vi "Offset Locking and Active Slave Locking v3.2.vi"() -> ()   [LabVIEW 2018]
uses:
  <vilib>/Utility/error.llb/DialogType.ctl
  <vilib>/Analysis/1siggen.llb/Ramp Pattern by Samples.vi
  <vilib>/measure/mamon.llb/Waveform Peak Detection for 1 Chan.vi
  <vilib>/addons/control/pid/pid.llb/PID Advanced (DBL).vi
  <vilib>/measure/NI_MAPro.lvlib
  <vilib>/addons/control/pid/NI_PID_pid.lvlib
  <vilib>/Analysis/NI_AALBase.lvlib
  <vilib>/measure/NI_MABase.lvlib
panel:
  in  "Drift Threshold":dbl
  out "Waveform Chart":dbl(graph)
  out "Slave Current Adj":dbl
  out "Master-Slave Peak Height":dbl
  in  "Locked Peak Height Min":dbl
  in  "Active Slave Lock On":bool
  in  "Slave Current Adjust":dbl
  out "Target \nPeak":dbl
  out "Calibration\n Peaks":dbl[](array[numeric])
  in  "Minimum \namplitude\nfor Calibration":dbl=2.1 format="%#_13g V"
  in  "width":i32=1000
  in  "start":dbl format="%0.2f"
  in  "end":dbl=1.0 format="%0.2f"
  in  "samples":i32=128
  in  "Waveform Test?":bool
  in  "reset signal":bool
  in  "phase":dbl format="%.2p"
  out "Chirp Rate":dbl format="%#_g GHz/ms"
  out "Single Mode?":bool
  out "# of Peaks found when Chirping?":i32
  in  "Minimum amplitude for Slave":dbl=0.15 format="%.2p"
  in  "Minimum \namplitude\nfor peaks":dbl=1.2 format="%#_13g V"
  in  "PZT Voltage to \nFrequency Conversion":dbl=-1.41655 format="%#_g V/GHz"
  out "PZT Chirp Output":waveform(dbl)(graph)
  in  "offset":dbl format="%0.2p V"
  in  "Sampling Info":cluster{"Fs":dbl, "#s":dbl}={"Fs"=10000.0, "#s"=100.0} {"Fs" format="%.2p"}
  in  "frequency":dbl=10.0 format="%0.2p Hz"
  in  "Chirp Amplitude":dbl=1.5 format="%0.2p GHz"
  in  "Run Chirp Program?":bool
  out "Run Time (min)":dbl
  out "standard deviation":dbl format="%0.3e"
  out "# found":i32
  out "Offset":dbl(graph)
  in  "Manual PZT Control":dbl format="%#_g V"
  in  "Engage PZT PID?":bool
  out "Offset (GHz)":dbl format="%#_4g"
  in  "# of Shots for Averaging":i32=100
  in  "Name Convention":string="Chirp Offset Lock Log"
  in  "Save Directory":path=path "C:/Users/LabUser/Google Drive/Measurements/04-2018"
  out "Enough\n peaks?":bool
  out "PZT Output":dbl(graph)
  in  "PID Gains":T1={"proportional gain (Kc)"=-1.0, "integral time (Ti, min)"=0.01, "derivative time (Td, min)"=0.0} {"derivative time (Td, min)" format="%.3f"; "integral time (Ti, min)" format="%.3f"; "proportional gain (Kc)" format="%.3f"}
  out "dt out (s)":dbl format="%.3f"
  in  "Frequency Offset Setpoint (GHz)":dbl=4.0 format="%.3f"
  out "GHz/sec":dbl
  out "dt":dbl format="%#_4g"
  out "Locations":dbl[](array[numeric]) format="%.2p"
  out "Amplitudes":dbl[](array[numeric]) format="%.2p"
  out "2nd Derivatives":dbl[](array[numeric]) format="%.2p"
  out "10 GHz FPI":dynamicdata(graph)
  in  "Stop":bool
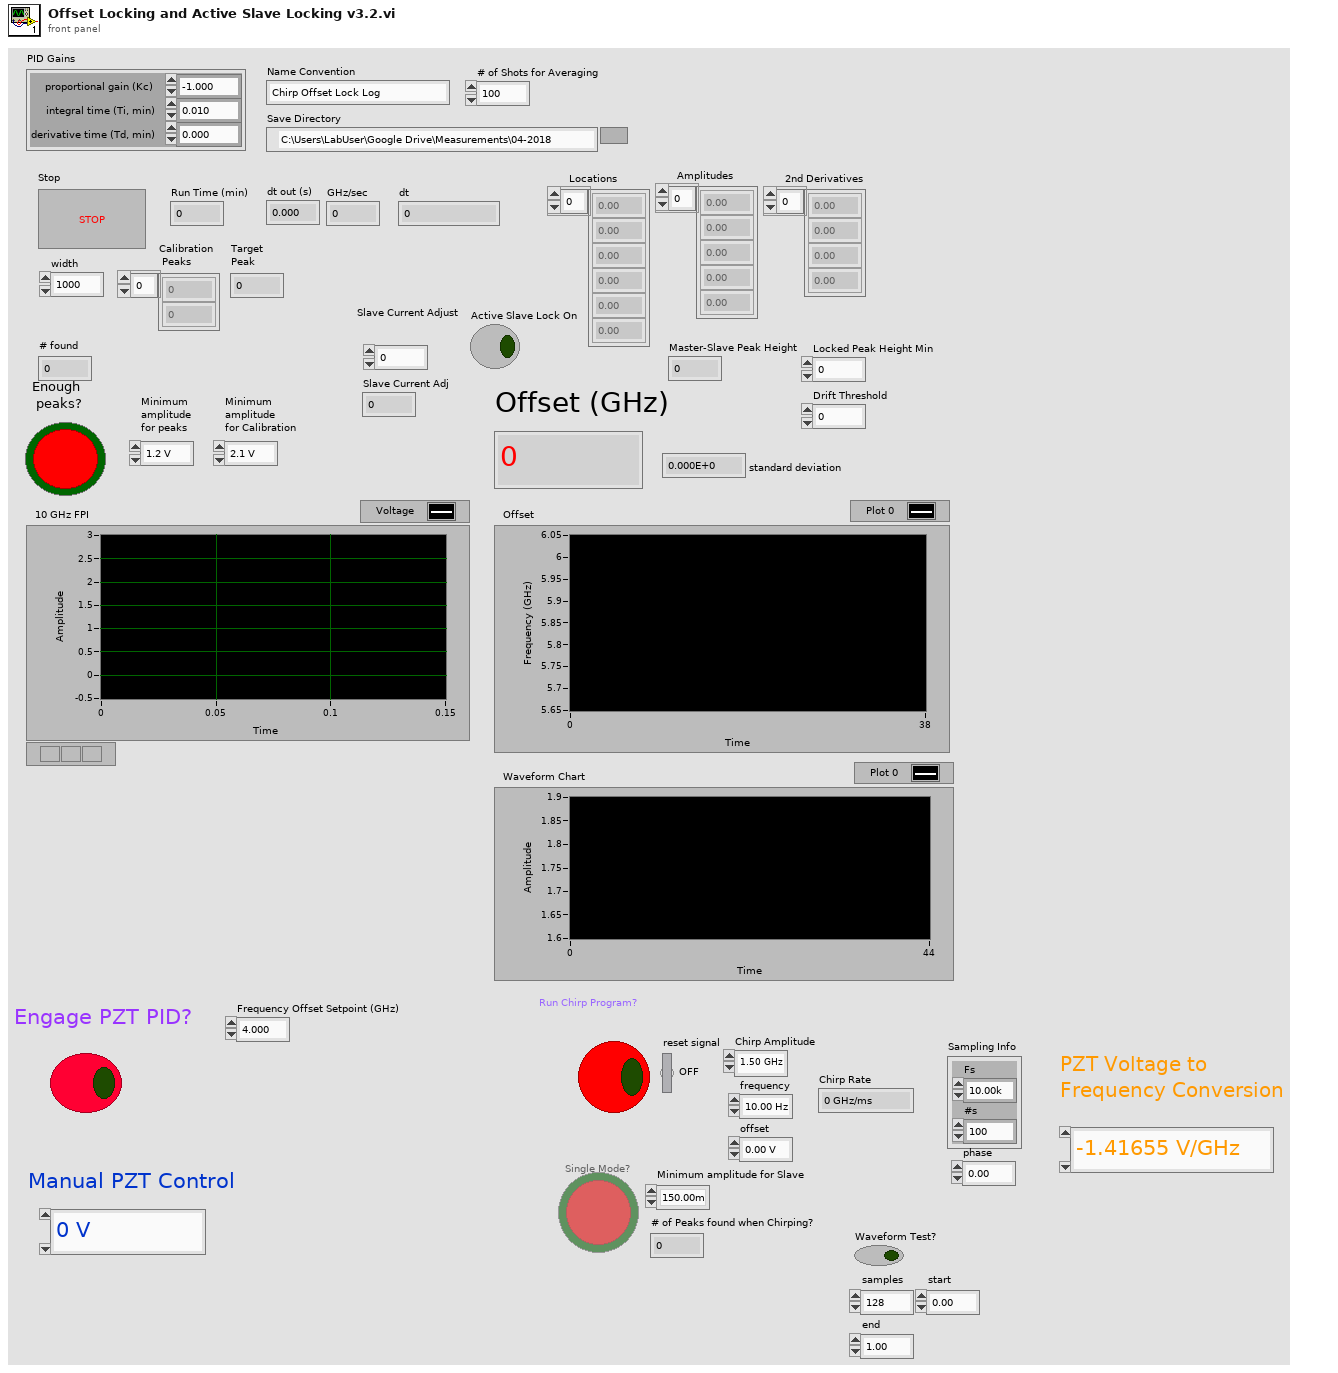
[diagram p1: front panel]
types:
  T1 = cluster{"proportional gain (Kc)":dbl, "integral time (Ti, min)":dbl, "derivative time (Td, min)":dbl}
  T2 = enum8{"Enabled", "Disabled", "Disabled and Grayed Out"}
  T3 = typedef "DialogType.ctl" = u16
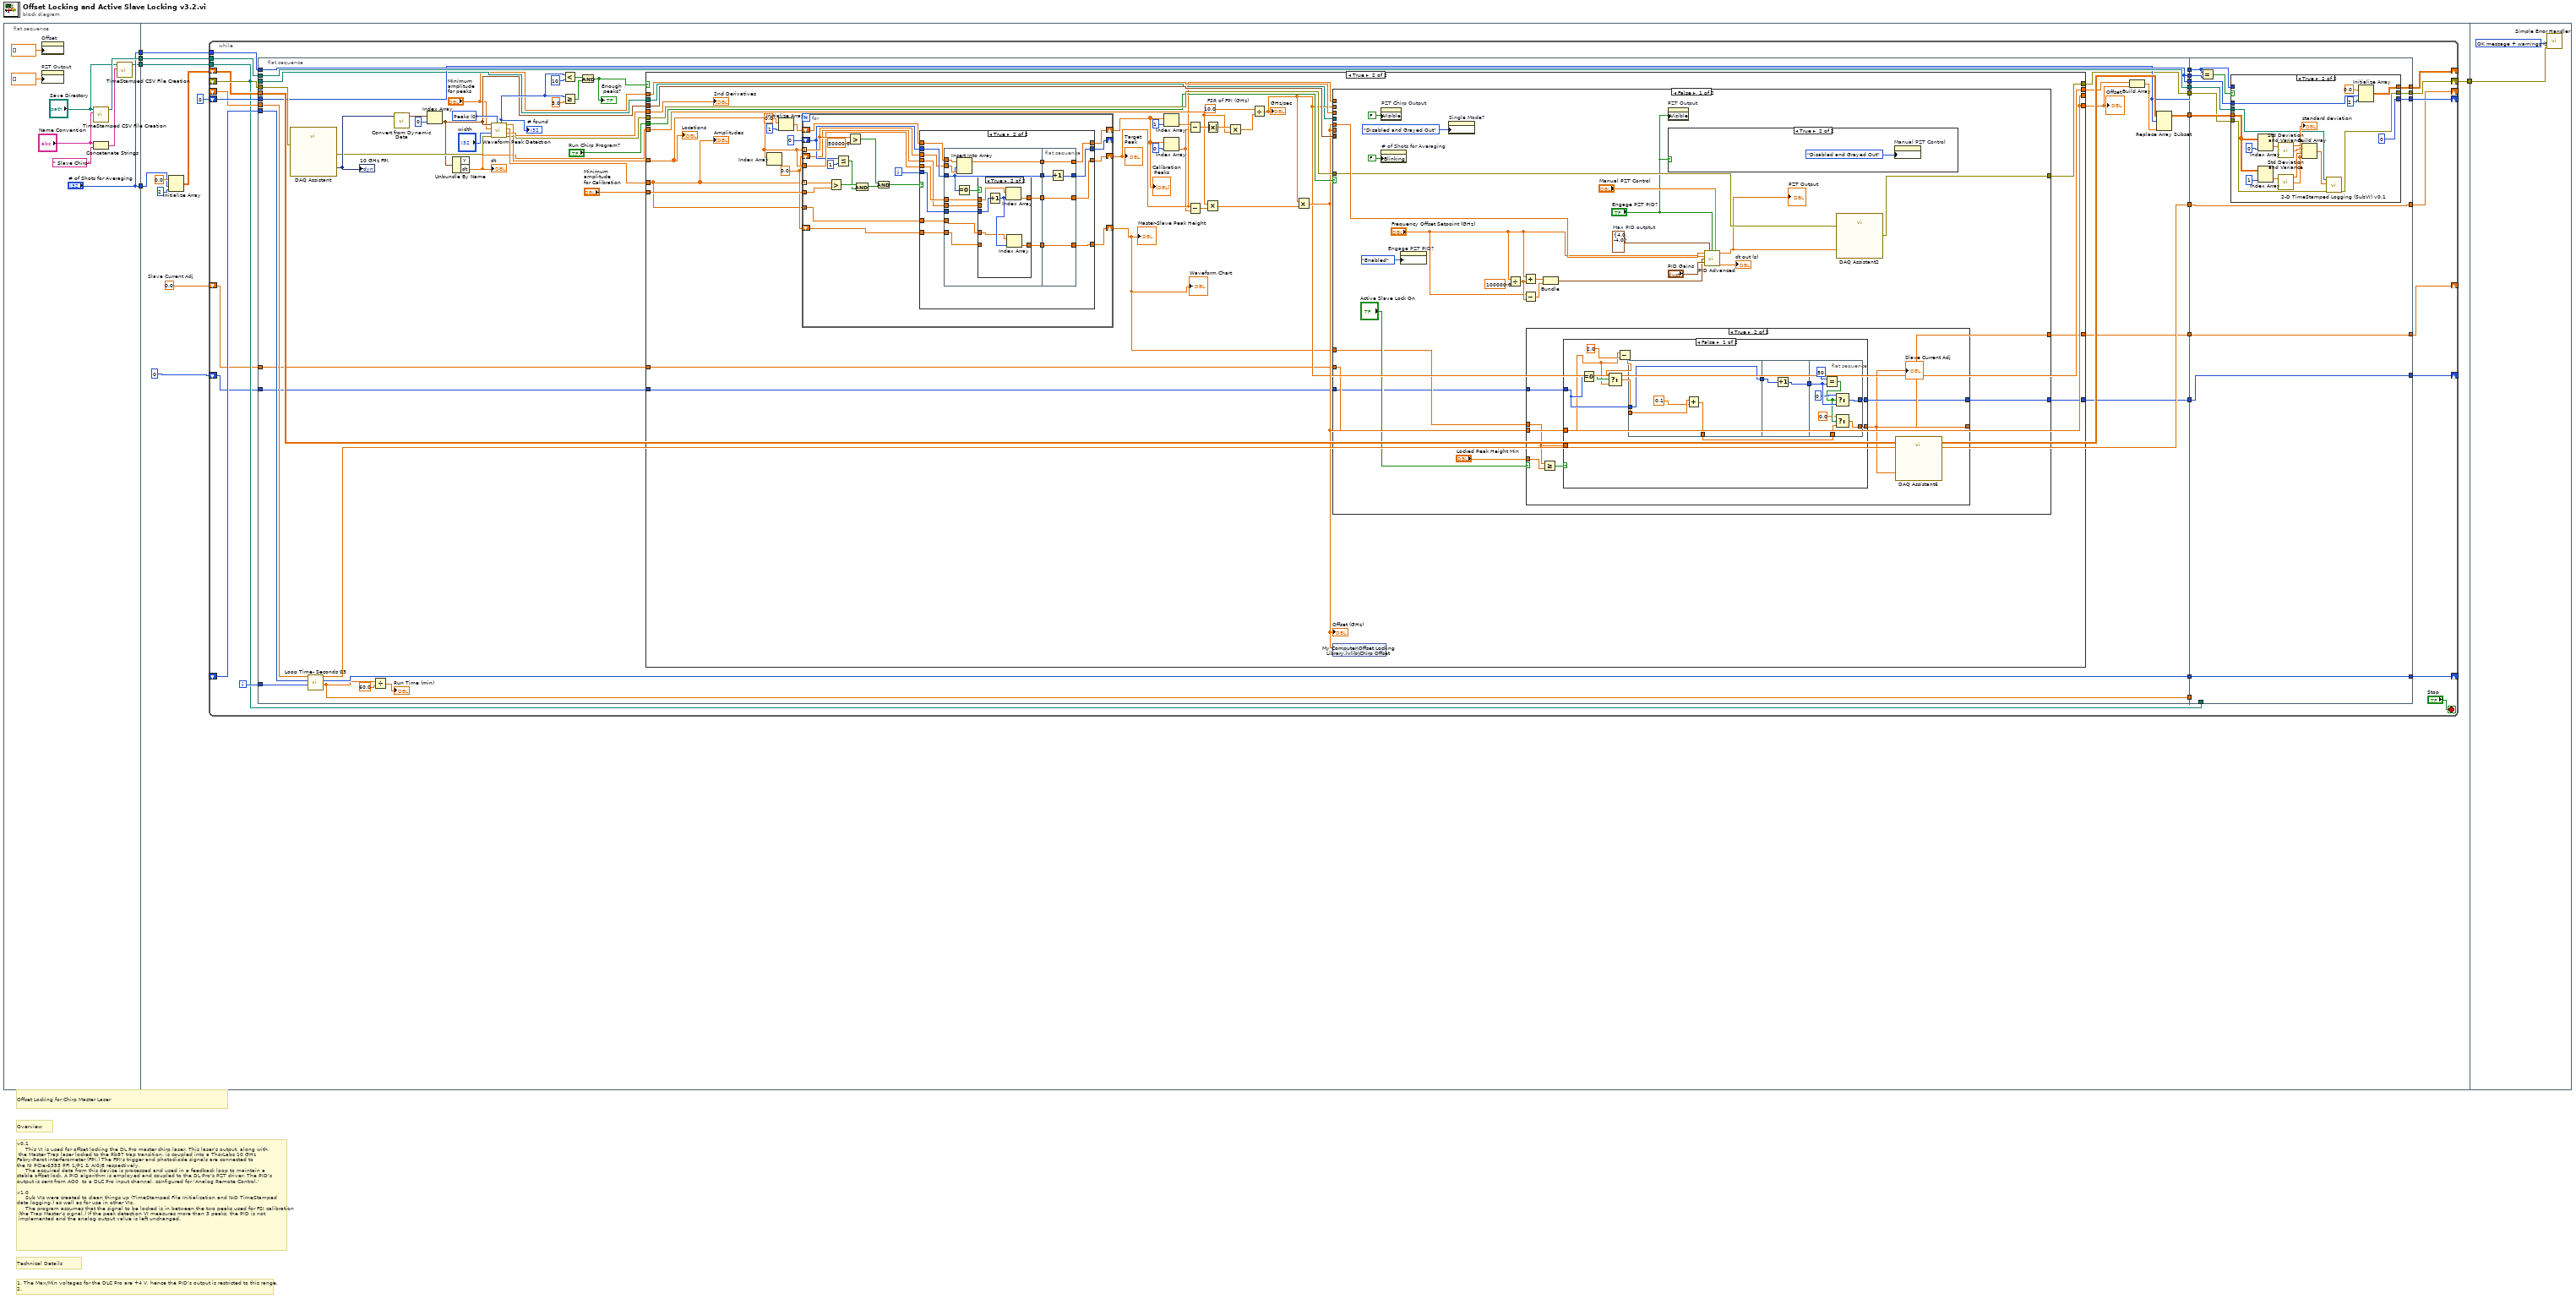
[diagram p0: block diagram]
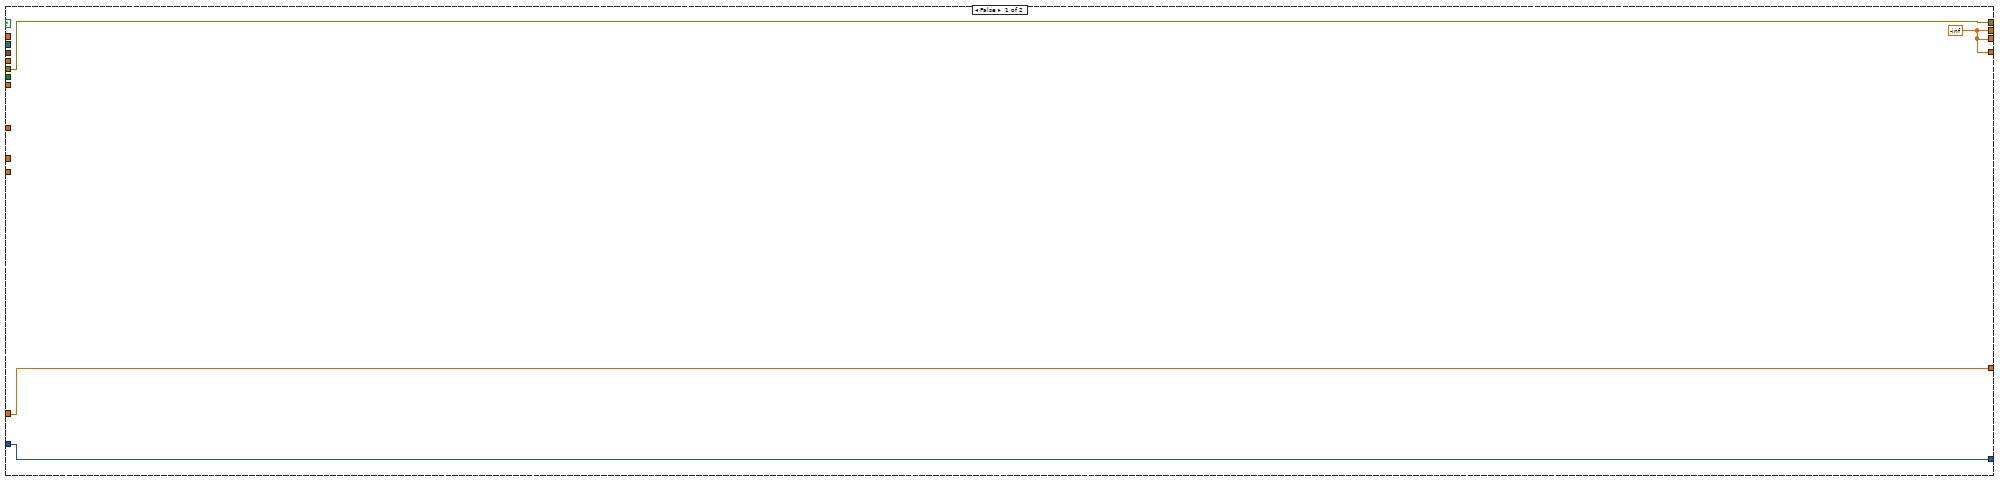
[diagram p2: hidden frame]
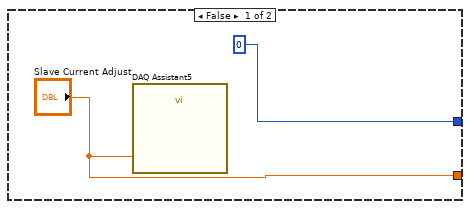
[diagram p5: hidden frame]
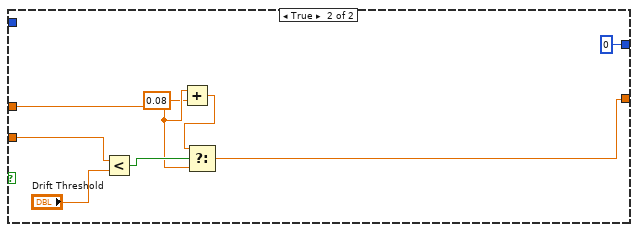
[diagram p6: hidden frame]
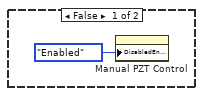
[diagram p7: hidden frame]
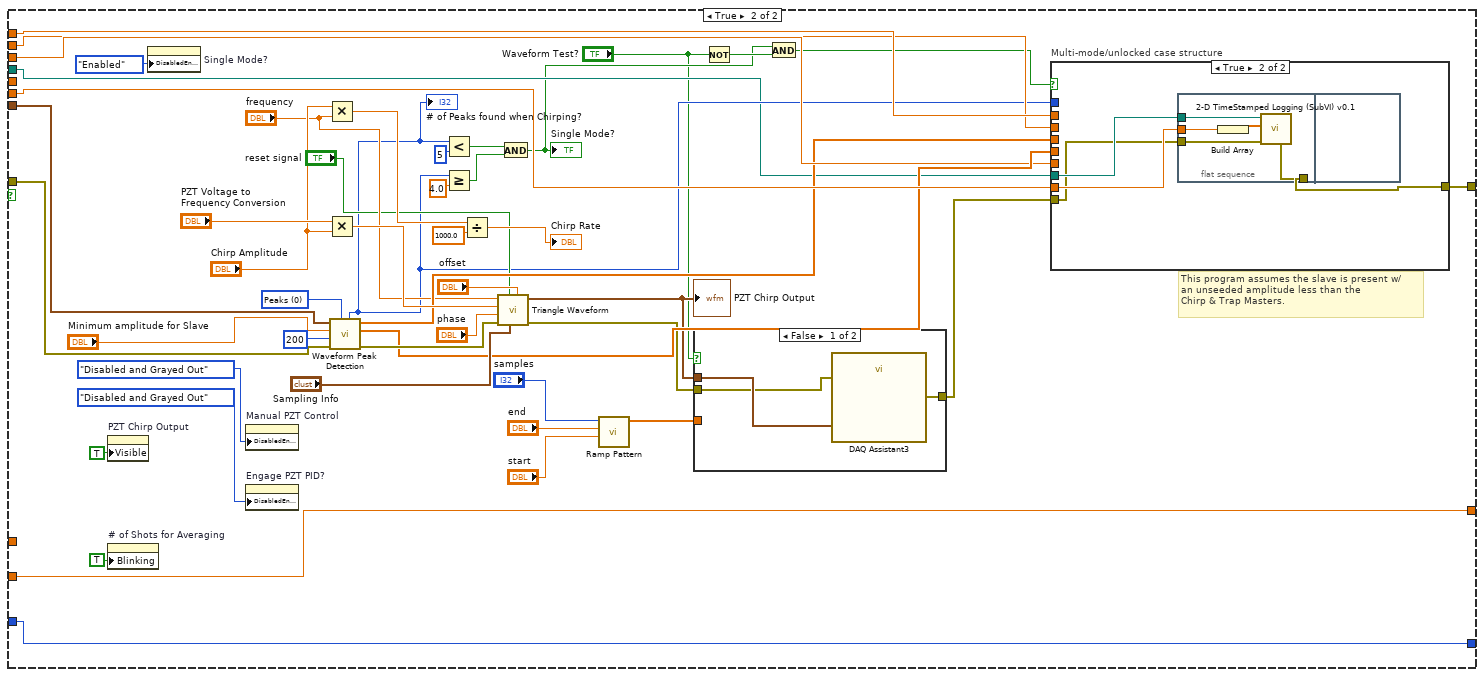
[diagram p8: hidden frame]
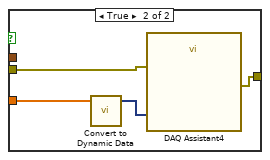
[diagram p9: hidden frame]
diagram:
  # "1. The Max/Min voltages for the DLC Pro are +4 V, hence the PID's output is restricted to this range.\n2."
  # "Technical Details"
  # "v0.1\n     This VI is used for offset locking the DL Pro master chirp laser. This laser's output, along with\n the Master Trap laser locked to the Rb87 trap transition, is coupled into a ThorLabs 10 GHz \nFabry-Perot interferometer (FPI.) The FPI's trigger and photodiode signals are connected to \nthe NI PCIe-6353 PFI 1/P1 & AI0/8 respectively. \n     The acquired data from this device is processed and used in a feedback loop to maintain a \nstable offset lock. A PID algorithm is employed and coupled to the DL Pro's PZT driver. The PID's\noutput is sent from AO0  to a DLC Pro input channel, configured for 'Analog Remote Control.'\n\nv1.0\n     Sub VIs were created to clean things up (TimeStamped File Initialization and N-D TimeStamped \ndata logging,) as well as for use in other VIs.\n     The program assumes that the signal to be locked is in between the two peaks used for FSI calibration\n (the Trap Master's signal.) If the peak detection VI measures more than 3 peaks, the PID is not\n implemented and the analog output value is left unchanged."
  # "Overview"
  # "Offset Locking for Chirp Master Laser"
  n1 = flat-sequence {
    tunnel: [w14] -> w5
    tunnel: ["# of Shots for Averaging"] -> w3
    tunnel: ["# of Shots for Averaging"] -> w2
    tunnel: [w6] -> w1
    tunnel: w5 -> [w25]
    tunnel: [w24] -> w4
    tunnel: w3 -> [w22]
    tunnel: w2 -> [w19]
    tunnel: w1 -> [w17]
    tunnel: w4 -> [w381]
    frame #0 {
      n2 = property on="Offset" class="WFChart (strict)"("History Data"=dbl[] []) -> ()  [unwired: 2 in, 2 out]
      n3 = property on="PZT Output" class="WFChart (strict)"("History Data"=dbl[] []) -> ()  [unwired: 2 in, 2 out]
      n4 = call "TimeStamped CSV File Creation.vi"("Name Convention"="Name Convention", "Save Directory"="Save Directory") -> ("path"=w14:path)  [unwired: 8 in, 1 out]
      n5 = Concatenate Strings("Name Convention", " Slave Chirp" ("string")) -> (w8:string)
      n6 = call "TimeStamped CSV File Creation.vi"("Name Convention"=w8, "Save Directory"="Save Directory") -> ("path"=w6:path)  [unwired: 8 in, 1 out]
    }
    frame #1 {
      w16 = 0.0  # Slave Current Adj
      n7 = Initialize Array(0.0 ("element"), w19, 2 ("dimension size")) -> (w21:dbl[][])
      n8 = while {
        shift-right: [w43] -> w24
        shift-left: _ -> [w54]
        tunnel: w25 -> [w52]
        shift-right: [w41] -> _
        shift-left: 0 -> [w50]
        tunnel: w22 -> [w48]
        shift-right: [w42] -> _
        shift-left: w21 -> [w45]
        shift-right: [w39] -> _
        shift-left: _ -> [w36]
        shift-right: [w37] -> _
        shift-left: _ -> [w35]
        tunnel: w17 -> [w32]
        shift-right: [w29] -> _
        shift-left: w16 -> [w31]
        shift-right: [w26] -> _
        shift-left: 0 -> [w28]
        i -> [w34]
        stop <- "Stop" stop-if-true
        n9 = flat-sequence {
          tunnel: w54 -> [w90]
          tunnel: [w66] -> w53
          tunnel: w52 -> [w88]
          tunnel: [w88] -> w51
          tunnel: w50 -> [w82]
          tunnel: [w82] -> w49
          tunnel: w48 -> [w83]
          tunnel: [w83] -> w47
          tunnel: [w87] -> w46
          tunnel: w45 -> [w86]
          tunnel: [w83] -> w44
          tunnel: [w81] -> w40
          tunnel: [w80] -> w38
          tunnel: w36 -> [w79]
          tunnel: w35 -> [w78]
          tunnel: w34 -> [w77]
          tunnel: [w69] -> w33
          tunnel: w32 -> [w63]
          tunnel: w31 -> [w59]
          tunnel: [w58] -> w30
          tunnel: w28 -> [w57]
          tunnel: [w56] -> w27
          tunnel: w53 -> [w354]
          tunnel: w51 -> [w355]
          tunnel: w49 -> [w349]
          tunnel: w47 -> [w359]
          tunnel: w46 -> [w356]
          tunnel: w44 -> [w357]
          tunnel: [w348] -> w43
          tunnel: [w353] -> w42
          tunnel: [w352] -> w41
          tunnel: w40 -> [w351]
          tunnel: [w351] -> w39
          tunnel: [w350] -> w37
          tunnel: w38 -> [w350]
          tunnel: w33 -> [_]
          tunnel: w32 -> [_]
          tunnel: w30 -> [w347]
          tunnel: [w347] -> w29
          tunnel: w27 -> [w346]
          tunnel: [w346] -> w26
          frame #0 {
            w92 = u16 0 items=["Peaks", "Valleys"] ("peaks/valleys")
            n10 = call "DAQ Assistant"("error in"=w90) -> ("data"=w97:dynamicdata, "error out"=w89:errorcluster)  [unwired: 16 in, 1 out]
            "10 GHz FPI" <- w97
            n11 = call "Loop Time- Seconds 03.vi"("Loop Iteration"=w77, "Shift Registered Time In"=w78, "Shift Registered In"=w79) -> ("t"=w69:dbl, "Shift Registered Time Out"=w80:u32, "Shift Registered Out"=w81:dbl)  [unwired: 6 in]
            n12 = Divide(x=w69, y=60.0) -> (x/y=→"Run Time (min)":dbl)
            n13 = call "Convert from Dynamic Data"("Dynamic Data Type"=w97) -> ("Array of Waveform"=w99:waveform(dbl)[])  [unwired: 3 in]
            n14 = Index Array(array=w99, index=0) -> (element=w64:waveform(dbl))
            n15 = Unbundle By Name(w64) -> ("dt"=w93:dbl)  [unwired: 1 out]
            "dt" <- w93
            n16 = call-poly <vilib>:"Waveform Peak Detection.vi"("peaks/valleys"=w92, "error in"=w89, "width"="width", "threshold"="Minimum \namplitude\nfor peaks", "Signal In"=w64) -> ("error out"=w67:errorcluster, "2nd Derivatives"=w95:dbl[], "Amplitudes"=w96:dbl[], "Locations"=w94:dbl[], "# found"=w74:i32)  [unwired: 2 in]
            "# found" <- w74
            n17 = Less?(x=w74, y=10) -> (x < y?=w72:bool)
            n18 = Greater Or Equal?(x=w74, y=3.0) -> (x >= y?=w75:bool)
            n19 = And(x=w72, y=w75) -> (x .and. y?=w71:bool)
            "Enough\n peaks?" <- w71
            n20 = case shown="True" w71 {
              tunnel: w96 -> [_ w109]
              tunnel: w95 -> [_ w138]
              tunnel: w94 -> [_ w117]
              tunnel: w93 -> [_ w132]
              tunnel: [w103 w124] -> w85
              tunnel: [w103 w126] -> w76
              tunnel: [w103 w126] -> _
              tunnel: w67 -> [w102 w130]
              tunnel: [w102 w129] -> w66
              tunnel: "Run Chirp Program?" -> [_ w128]
              tunnel: w64 -> [_ w127]
              tunnel: "Minimum \namplitude\nfor peaks" -> [_ w125]
              tunnel: w63 -> [_ w123]
              tunnel: "Minimum \namplitude\nfor Calibration" -> [_ w122]
              tunnel: w59 -> [w101 w108]
              tunnel: [w101 w107] -> w58
              tunnel: w57 -> [w100 w106]
              tunnel: [w100 w105] -> w56
              frame False {
                w103 = -inf
              }
              frame True {
                w110 = 0.0
                w137 = 10.0  # FSR of FPI (GHz)
                n21 = Index Array(array=w117) -> ()  [unwired: 1 in, 1 out]
                n22 = Initialize Array(0.0 ("element"), 1 ("dimension size")) -> (w118:dbl[])
                n23 = for {
                  tunnel: w117 -> [w149] mode=indexing
                  tunnel: w109 -> [w142] mode=indexing
                  tunnel: w122 -> [w154]
                  shift-right: [w145] -> w116
                  shift-left: w118 -> [w159]
                  shift-right: [w158] -> _
                  shift-left: 0 -> [w146]
                  shift-right: [w144] -> w112
                  shift-left: w110 -> [w143]
                  tunnel: w117 -> [w147]
                  shift-right: [w140] -> w104
                  shift-left: w110 -> [w141]
                  tunnel: w109 -> [w139]
                  i -> [w148]
                  n24 = Greater?(x=w142, y=w154) -> (0:w157:bool)
                  n25 = Less Or Equal?(x=w146, y=1) -> (x <= y?=w155:bool)
                  n26 = Greater?(x=w149, y=50000.0) -> (0:w152:bool)
                  n27 = And(x=w157, y=w155) -> (x .and. y?=w153:bool)
                  n28 = And(x=w152, y=w153) -> (x .and. y?=w150:bool)
                  n29 = case shown="True" w150 {
                    tunnel: w159 -> [w162 w179]
                    tunnel: w146 -> [w163 w178]
                    tunnel: [w163 w175] -> w158
                    tunnel: w149 -> [_ w177]
                    tunnel: w148 -> [_ w172]
                    tunnel: w147 -> [_ w171]
                    tunnel: [w162 w173] -> w145
                    tunnel: [w161 w169] -> w144
                    tunnel: w143 -> [w161 w168]
                    tunnel: w141 -> [w160 w167]
                    tunnel: [w160 w164] -> w140
                    tunnel: w139 -> [_ w166]
                    frame False {
                    }
                    frame True {
                      n30 = flat-sequence {
                        tunnel: w179 -> [w191]
                        tunnel: w178 -> [w188]
                        tunnel: w177 -> [w190]
                        tunnel: [w189] -> w176
                        tunnel: [w188] -> w174
                        tunnel: w172 -> [w185]
                        tunnel: w171 -> [w187]
                        tunnel: [w186] -> w170
                        tunnel: w168 -> [w183]
                        tunnel: w167 -> [w180]
                        tunnel: w166 -> [w182]
                        tunnel: [w181] -> w165
                        tunnel: w176 -> [w202]
                        tunnel: [w204] -> w175
                        tunnel: w174 -> [w203]
                        tunnel: [w202] -> w173
                        tunnel: w170 -> [w201]
                        tunnel: [w201] -> w169
                        tunnel: w165 -> [w200]
                        tunnel: [w200] -> w164
                        frame #0 {
                          n31 = Equal To 0?(x=w188) -> (x = 0?=w184:bool)
                          n32 = Insert Into Array(array=w191, index=w188, new element=w190) -> (w189:dbl[])
                          n33 = case shown="True" w184 {
                            tunnel: w187 -> [_ w199]
                            tunnel: [w193 w198] -> w186
                            tunnel: w185 -> [_ w197]
                            tunnel: w183 -> [w193 _]
                            tunnel: w182 -> [_ w195]
                            tunnel: [w192 w194] -> w181
                            tunnel: w180 -> [w192 _]
                            frame False {
                            }
                            frame True {
                              n34 = Increment(x=w197) -> (x+1=w196:i32)
                              n35 = Index Array(array=w199, index=w196) -> (element=w198:dbl)
                              n36 = Index Array(array=w195, index=w196) -> (element=w194:dbl)
                            }
                          }
                        }
                        frame #1 {
                          n37 = Increment(x=w203) -> (x+1=w204:i32)
                        }
                      }
                    }
                  }
                }
                "Calibration\n Peaks" <- w116
                "Target \nPeak" <- w112
                "Master-Slave Peak Height" <- w104
                "Waveform Chart" <- w104
                n38 = Index Array(array=w116, index=1) -> (element=w113:dbl)
                n39 = Index Array(array=w116, index=0) -> (element=w111:dbl)
                n40 = Subtract(x=w113, y=w111) -> (x-y=w135:dbl)
                n41 = Subtract(x=w112, y=w111) -> (x-y=w133:dbl)
                n42 = Multiply(x=w132, y=w133) -> (x*y=w131:dbl)
                n43 = Absolute Value(x=w135) -> (abs(x)=w134:dbl)
                n44 = Multiply(x=w134, y=w132) -> (x*y=w136:dbl)
                n45 = Divide(x=w137, y=w136) -> (x/y=w124:dbl)
                "GHz/sec" <- w124
                n46 = Multiply(x=w124, y=w131) -> (x*y=w126:dbl)
                "Offset (GHz)" <- w126
                n47 = case shown="False" w128 {
                  tunnel: w126 -> [w226 _]
                  tunnel: w130 -> [w225 w312]
                  tunnel: [w224 w285] -> w129
                  tunnel: w127 -> [_ w313]
                  tunnel: w126 -> [_ w309]
                  tunnel: w125 -> [_ w303]
                  tunnel: w112 -> [_ w301]
                  tunnel: w124 -> [_ w300]
                  tunnel: w123 -> [_ w287]
                  tunnel: w104 -> [w209 _]
                  tunnel: w108 -> [w208 w276]
                  tunnel: [w207 w276] -> w107
                  tunnel: w106 -> [w206 w275]
                  tunnel: [w205 w275] -> w105
                  frame False {
                    w228 = cluster{"output high":dbl, "output low":dbl} {"output high"=4.0, "output low"=-4.0}  # Max PID outptut
                    n48 = property on="PZT Chirp Output" class="WFGraph (strict)"("Visible"=FALSE) -> ()  [unwired: 2 in, 2 out]
                    n49 = property on="# of Shots for Averaging" class="DigNum (strict)"("Blinking"=FALSE) -> ()  [unwired: 2 in, 2 out]
                    n50 = property on="Engage PZT PID?" class="Bool (strict)"("DisabledEnum"=T2."Enabled" ("Disabled")) -> ()  [unwired: 2 in, 2 out]
                    n51 = property on="Single Mode?" class="Bool (strict)"("DisabledEnum"=T2."Disabled and Grayed Out" ("Disabled")) -> ()  [unwired: 2 in, 2 out]
                    n52 = Divide(x="Frequency Offset Setpoint (GHz)", y=100000.0) -> (x/y=w216:dbl)
                    n53 = Add(x="Frequency Offset Setpoint (GHz)", y=w216) -> (x+y=w214:dbl)
                    n54 = Subtract(x="Frequency Offset Setpoint (GHz)", y=w216) -> (x-y=w213:dbl)
                    n55 = case shown="True" "Active Slave Lock On" {
                      tunnel: ["Slave Current Adjust" w233] -> w207
                      tunnel: "Locked Peak Height Min" -> [_ w237]
                      tunnel: w209 -> [_ w234]
                      tunnel: w208 -> [_ w238]
                      tunnel: w206 -> [_ w236]
                      tunnel: [0 ("t") w235] -> w205
                      frame False {
                        n56 = call "DAQ Assistant5"("data"="Slave Current Adjust") -> ()  [unwired: 17 in, 2 out]
                      }
                      frame True {
                        n57 = Greater Or Equal?(x=w234, y=w237) -> (x >= y?=w239:bool)
                        n58 = case shown="False" w239 {
                          tunnel: w238 -> [w243 w267]
                          tunnel: [w241 w268] -> w233
                          tunnel: w236 -> [w246 _]
                          tunnel: [w247 0 ("t")] -> w235
                          tunnel: w234 -> [_ w271]
                          frame False {
                            n59 = Equal To 0?(x=w246) -> (x = 0?=w245:bool)
                            n60 = Subtract(x=w243, y=2.0) -> (x-y=w244:dbl)
                            n61 = Select(t=w244, s=w245, f=w243) -> (s? t:f=w242:dbl)
                            n62 = flat-sequence {
                              tunnel: w242 -> [w254]
                              tunnel: w246 -> [w252]
                              tunnel: [w253] -> w240
                              tunnel: [w252] -> w249
                              tunnel: w249 -> [w256]
                              tunnel: [w255] -> w248
                              tunnel: w248 -> [w263]
                              tunnel: [w261] -> w247
                              tunnel: w240 -> [w259]
                              tunnel: [w258] -> w241
                              frame #0 {
                                n63 = Add(x=w254, y=0.1 ("x")) -> (x+y=w253:dbl)
                              }
                              frame #1 {
                                n64 = Increment(x=w256) -> (x+1=w255:i32)
                              }
                              frame #2 {
                                n65 = Equal?(x=50, y=w263) -> (x = y?=w260:bool)
                                n66 = Select(t=0, s=w260, f=w263) -> (s? t:f=w261:i32)
                                n67 = Select(t=0.0, s=w260, f=w259) -> (s? t:f=w258:dbl)
                              }
                            }
                          }
                          frame True {
                            n68 = Less?(x=w271, y="Drift Threshold") -> (x < y?=w269:bool)
                            n69 = Add(x=w267, y=0.08) -> (x+y=w265:dbl)
                            n70 = Select(t=w265, s=w269, f=w267) -> (s? t:f=w268:dbl)
                          }
                        }
                        "Slave Current Adj" <- w233
                        n71 = call "DAQ Assistant6"("data"=w233) -> ()  [unwired: 17 in, 2 out]
                      }
                    }
                    n72 = Bundle(w214, w213) -> (w212:cluster{dbl, dbl})  [unwired: 1 in]
                    n73 = property on="PZT Output" class="WFChart (strict)"("Visible"="Engage PZT PID?") -> ()  [unwired: 2 in, 2 out]
                    n74 = case shown="True" "Engage PZT PID?" {
                      frame False {
                        n75 = property on="Manual PZT Control" class="DigNum (strict)"("DisabledEnum"=T2."Enabled" ("Disabled")) -> ()  [unwired: 2 in, 2 out]
                      }
                      frame True {
                        n76 = property on="Manual PZT Control" class="DigNum (strict)"("DisabledEnum"=T2."Disabled and Grayed Out" ("Disabled")) -> ()  [unwired: 2 in, 2 out]
                      }
                    }
                    n77 = call-poly <vilib>:"PID Advanced.vi"("setpoint"="Frequency Offset Setpoint (GHz)", "output range"=w228, "auto? (T)"="Engage PZT PID?", "manual control"="Manual PZT Control", "process variable"=w226, "setpoint range"=w212, "PID gains"="PID Gains") -> ("output"=w223:dbl, "dt out (s)"=→"dt out (s)":dbl)  [unwired: 7 in]
                    "PZT Output" <- w223
                    n78 = call "DAQ Assistant2"("data"=w223, "error in"=w225) -> ("error out"=w224:errorcluster)  [unwired: 16 in, 1 out]
                  }
                  frame True {
                    w299 = u16 0 items=["Peaks", "Valleys"] ("peaks/valleys")
                    # "This program assumes the slave is present w/ \nan unseeded amplitude less than the \nChirp & Trap Masters."
                    n79 = property on="PZT Chirp Output" class="WFGraph (strict)"("Visible"=TRUE) -> ()  [unwired: 2 in, 2 out]
                    n80 = property on="# of Shots for Averaging" class="DigNum (strict)"("Blinking"=TRUE) -> ()  [unwired: 2 in, 2 out]
                    n81 = property on="Single Mode?" class="Bool (strict)"("DisabledEnum"=T2."Enabled" ("Disabled")) -> ()  [unwired: 2 in, 2 out]
                    n82 = property on="Manual PZT Control" class="DigNum (strict)"("DisabledEnum"=T2."Disabled and Grayed Out" ("Disabled")) -> ()  [unwired: 2 in, 2 out]
                    n83 = property on="Engage PZT PID?" class="Bool (strict)"("DisabledEnum"=T2."Disabled and Grayed Out" ("Disabled")) -> ()  [unwired: 2 in, 2 out]
                    n84 = Multiply(x="Chirp Amplitude", y="frequency") -> (x*y=w294:dbl)
                    n85 = Multiply(x="PZT Voltage to \nFrequency Conversion", y="Chirp Amplitude") -> (x*y=w315:dbl)
                    n86 = call-poly <vilib>:"Waveform Peak Detection.vi"("peaks/valleys"=w299, "error in"=w312, "width"=200, "threshold"="Minimum amplitude for Slave", "Signal In"=w313) -> ("error out"=w311:errorcluster, "Amplitudes"=w304:dbl[], "Locations"=w302:dbl[], "# found"=w288:i32)  [unwired: 2 in, 1 out]
                    "# of Peaks found when Chirping?" <- w288
                    n87 = Less?(x=w288, y=5) -> (x < y?=w305:bool)
                    n88 = Greater Or Equal?(x=w288, y=4.0) -> (x >= y?=w307:bool)
                    n89 = Divide(x=w294, y=1000.0) -> (x/y=→"Chirp Rate":dbl)
                    n90 = call <vilib>:"Triangle Waveform.vi"("offset"="offset", "sampling info"="Sampling Info", "reset signal"="reset signal", "error in (no error)"=w311, "phase"="phase", "amplitude"=w315, "frequency"="frequency") -> ("error out"=w289:errorcluster, "signal out"=w290:waveform(dbl))  [unwired: 3 in]
                    "PZT Chirp Output" <- w290
                    n91 = And(x=w305, y=w307) -> (x .and. y?=w283:bool)
                    "Single Mode?" <- w283
                    n92 = call-poly <vilib>:"Ramp Pattern.vi"("start"="start", "end"="end", "samples"="samples") -> ("Ramp Pattern"=w280:dbl[])  [unwired: 7 in, 1 out]
                    n93 = case shown="False" "Waveform Test?" {
                      tunnel: w290 -> [w325 _]
                      tunnel: w289 -> [w324 w329]
                      tunnel: [w323 w328] -> w286
                      tunnel: w280 -> [_ w327]
                      frame False {
                        n94 = call "DAQ Assistant3"("data"=w325, "error in"=w324) -> ("error out"=w323:errorcluster)  [unwired: 16 in, 1 out]
                      }
                      frame True {
                        n95 = call "Convert to Dynamic Data"("Array"=w327) -> ("Dynamic Data Type"=w326:dynamicdata)  [unwired: 3 in]
                        n96 = call "DAQ Assistant4"("data"=w326, "error in"=w329) -> ("error out"=w328:errorcluster)  [unwired: 16 in, 1 out]
                      }
                    }
                    n97 = Not(x="Waveform Test?") -> (.not. x?=w284:bool)
                    n98 = And(x=w283, y=w284) -> (x .and. y?=w282:bool)
                    n99 = case "Multi-mode/unlocked case structure" shown="True" w282 {
                      tunnel: w309 -> [_ w340]
                      tunnel: w288 -> [w336 _]
                      tunnel: w304 -> [w335 _]
                      tunnel: w303 -> [w334 _]
                      tunnel: w302 -> [w333 _]
                      tunnel: w301 -> [w332 _]
                      tunnel: w300 -> [w331 _]
                      tunnel: w287 -> [_ w339]
                      tunnel: w286 -> [w330 w338]
                      tunnel: [w330 w337] -> w285
                      frame False {
                        n100 = for {
                          N: w336 -> [_]
                          tunnel: w335 -> [_] mode=indexing
                          tunnel: w334 -> [_]
                          tunnel: w333 -> [_] mode=indexing
                          tunnel: w332 -> [_]
                          tunnel: w331 -> [_]
                        }
                      }
                      frame True {
                        n101 = flat-sequence {
                          tunnel: w340 -> [w345]
                          tunnel: w339 -> [w343]
                          tunnel: w338 -> [w342]
                          tunnel: [w341] -> w337
                          frame #0 {
                            n102 = Build Array(w345) -> (w344:dbl[])
                            n103 = call "2-D TimeStamped Logging (SubVI) v0.1.vi"("error in (no error)"=w342, "array"=w344, "path"=w343) -> ("error out"=w341:errorcluster)  [unwired: 8 in]
                          }
                          frame #1 {
                          }
                        }
                      }
                    }
                  }
                }
                n104 = shared-variable "My Computer\\Offset Locking Library.lvlib\\Chirp Offset"(w126) -> ()  [unwired: 1 in, 1 out]
                "2nd Derivatives" <- w138
                "Amplitudes" <- w109
                "Locations" <- w117
              }
            }
            "Offset" <- w76
            n105 = Build Array(w85, w76) -> (w84:dbl[])
            n106 = Replace Array Subset(array=w86, new element=w84, index (row)=w82) -> (w87:dbl[][])  [unwired: 1 in]
          }
          frame #1 {
            n107 = Equal?(x=w349, y=w359) -> (x = y?=w358:bool)
            n108 = case shown="True" w358 {
              tunnel: w357 -> [_ w363]
              tunnel: w356 -> [w362 w376]
              tunnel: w355 -> [_ w370]
              tunnel: w354 -> [w360 w369]
              tunnel: [w362 w366] -> w353
              tunnel: w349 -> [w361 _]
              tunnel: [w361 0] -> w352
              tunnel: [w360 w364] -> w348
              frame False {
              }
              frame True {
                n109 = Index Array(array=w376, index (col)=0 ("disabled index (col)")) -> (element=w379:dbl[])  [unwired: 1 in]
                n110 = Index Array(array=w376, index (col)=1 ("disabled index (col)")) -> (element=w377:dbl[])  [unwired: 1 in]
                n111 = call <vilib>:"Std Deviation and Variance.vi"("X"=w379) -> ("mean"=w375:dbl, "standard deviation"=w374:dbl)  [unwired: 1 in, 1 out]
                n112 = call <vilib>:"Std Deviation and Variance.vi"("X"=w377) -> ("mean"=w373:dbl, "standard deviation"=w372:dbl)  [unwired: 1 in, 1 out]
                "standard deviation" <- w372
                n113 = Build Array(w375, w374, w373, w372) -> (w371:dbl[])
                n114 = call "2-D TimeStamped Logging (SubVI) v0.1.vi"("error in (no error)"=w369, "array"=w371, "path"=w370) -> ("error out"=w364:errorcluster)  [unwired: 8 in]
                n115 = Initialize Array(0.0 ("element"), w363, 2 ("dimension size")) -> (w366:dbl[][])
              }
            }
          }
        }
      }
    }
    frame #2 {
      w382 = T3 3 items=["no dialog", "OK message", "continue or stop message", "OK message + warnings", "continue/stop + warnings"] ("type of dialog (OK msg:1)")
      n116 = call <vilib>:"Simple Error Handler.vi"("type of dialog (OK msg:1)"=w382, "error in (no error)"=w381) -> ()  [unwired: 3 in, 5 out]
    }
  }
